vi "GetIntFromNode(viaStringNodePath).vi"(2 "Path":string, 3 "error in":errorcluster, 5 "Tree DVR in":refnum<data-value>) -> (0 "error out":errorcluster, 1 "Int32":i32)   [LabVIEW 2014]
uses:
  <vilib>/MDSplus/Classes/Tree_Class/Tree.lvclass
  <vilib>/MDSplus/Library/MDSplus.lvlib
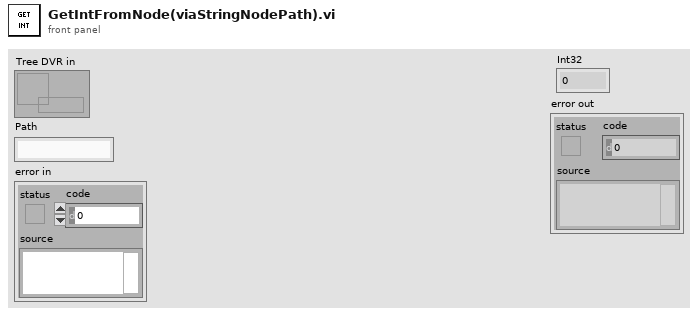
[diagram p1: front panel]
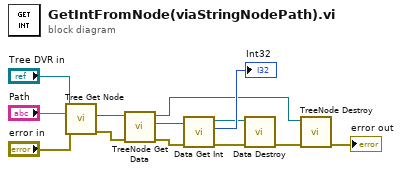
[diagram p0: block diagram]
diagram:
  n1 = call <vilib>:"Tree Get Node.vi"("error in (no error)"="error in", "Path"="Path", "Tree DVR in"="Tree DVR in") -> ("error out"=w12:errorcluster, "Node out"=w13:refnum<data-value>)  [unwired: 6 in, 1 out]
  n2 = call <vilib>:"TreeNode Get Data.vi"("error in (no error)"=w12, "TreeNode DVR in"=w13) -> ("error out"=w11:errorcluster, "Data out"=w10:refnum<data-value>, "TreeNode DVR out"=w3:refnum<data-value>)  [unwired: 7 in]
  n3 = call <vilib>:"Data Get Int.vi"("error in (no error)"=w11, "Data DVR in"=w10) -> ("error out"=w6:errorcluster, "I32 out"=→"Int32":i32, "Data DVR out"=w4:refnum<data-value>)  [unwired: 7 in]
  n4 = call <vilib>:"Data Destroy.vi"("error in (no error)"=w6, "Data DVR in"=w4) -> ("error out"=w5:errorcluster)  [unwired: 9 in]
  n5 = call <vilib>:"TreeNode Destroy.vi"("error in (no error)"=w5, "TreeNode DVR in"=w3) -> ("error out"=→"error out":errorcluster)  [unwired: 9 in]
